vi "Turn on Display.vi"(6 "chip select  (1st chip)":enum16{"1st chip", "2nd chip"}(ring), 8 "error in (no error)":errorcluster, 9 "cursor option":T1(ring)=enum."cursor on & no blink", 10 "display on?":bool=TRUE, 11 "LCD in":refnum<class "Character LCD.lvclass">) -> (0 "error out":errorcluster, 3 "LCD out":refnum<class "Character LCD.lvclass">)   [LabVIEW 2015, in "HD44780 Host.lvlib"]
uses:
  HD44780 Host.lvlib
  Internal/LCD Class/Character LCD.lvclass
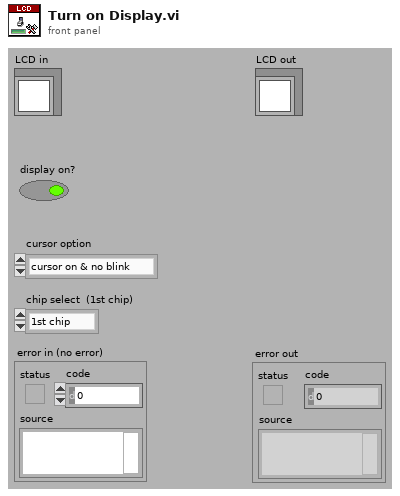
[diagram p1: front panel]
types:
  T1 = enum8{"cursor off", "cursor on & no blink", "cursor on & blink"}
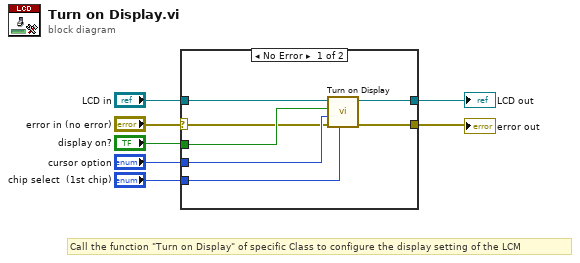
[diagram p0: block diagram]
diagram:
  # "Call the function \"Turn on Display\" of specific Class to configure the display setting of the LCM"
  n1 = case shown="No Error" "error in (no error)" {
    selector: "error in (no error)" -> [w8 w16]
    tunnel: [w9 w16] -> w7
    tunnel: "display on?" -> [w14 _]
    tunnel: "cursor option" -> [w13 _]
    tunnel: "chip select  (1st chip)" -> [w12 _]
    tunnel: "LCD in" -> [w11 w15]
    tunnel: [w10 w15] -> w1
    frame No Error {
      n2 = call-dynamic "Turn on Display.vi"("chip select  (1st chip)"=w12, "error in (no error)"=w8, "cursor option"=w13, "display on?"=w14, "Character LCD in"=w11) -> ("error out"=w9:errorcluster, "Character LCD out"=w10:refnum<class "Character LCD.lvclass">)  [unwired: 5 in]
    }
    frame Error {
    }
  }
  "error out" <- w7
  "LCD out" <- w1
